vi "SaveHighscores.vi"(8 "error in (no error)":errorcluster, 11 "Highscore in":refnum<class "Highscore.lvclass">) -> (0 "error out":errorcluster, 3 "Highscore out":refnum<class "Highscore.lvclass">)   [LabVIEW 2019, in "RT_Game.lvlib" / "Highscore.lvclass"]
uses:
  Highscore.lvclass
  Highscore.lvclass/Highscore.ctl
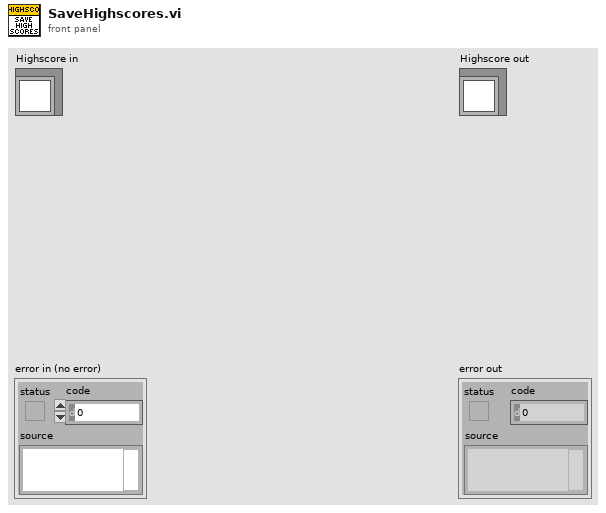
[diagram p1: front panel]
types:
  T1 = enum16{"open", "replace", "create", "open or create", "replace or create", "replace or create with confirmation"}
  T2 = typedef "RT_Game.lvlib/Highscore.lvclass/HighscoreEntry.ctl" = cluster{"Name":string, "Score":dbl}
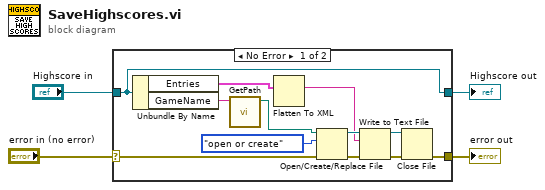
[diagram p0: block diagram]
diagram:
  n1 = case shown="No Error" "error in (no error)" {
    selector: "error in (no error)" -> [w16 w18]
    tunnel: [w9 w18] -> w3
    tunnel: [w14 w17] -> w1
    tunnel: "Highscore in" -> [w14 w17]
    frame No Error {
      n2 = Unbundle By Name(w14) -> ("Entries"=w5:T2[], "GameName"=w13:string)
      n3 = call "GetPath.vi"("GameName"=w13) -> ("appended path"=w12:path)  [unwired: 10 in]
      n4 = Flatten To XML(anything=w5) -> (xml string=w6:string)
      n5 = Open/Create/Replace File(file path (use dialog)=w12, error in=w16, operation (0:open)=T1."open or create") -> (refnum out=w8:refnum<file>, error out=w15:errorcluster)  [unwired: 3 in, 1 out]
      n6 = Write to Text File(file (use dialog)=w8, text=w6, error in=w15) -> (refnum out=w7:refnum<file>, error out=w10:errorcluster)  [unwired: 1 in, 1 out]
      n7 = Close File(refnum=w7, error in=w10) -> (error out=w9:errorcluster)  [unwired: 1 out]
    }
    frame Error {
    }
  }
  "error out" <- w3
  "Highscore out" <- w1
